vi "顺序结构.vi"() -> ()   [LabVIEW 2017]
panel:
  out "布尔":bool
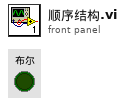
[diagram p1: front panel]
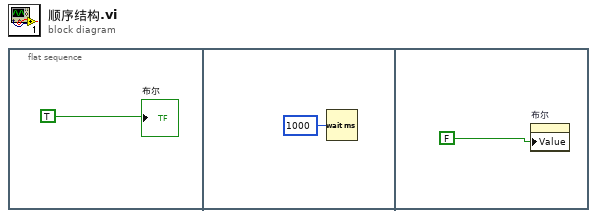
[diagram p0: block diagram]
diagram:
  n1 = flat-sequence {
    frame #0 {
      "布尔" <- TRUE
    }
    frame #1 {
      n2 = Wait (ms)(milliseconds to wait=u32 1000 ("等待时间（毫秒）")) -> ()  [unwired: 1 out]
    }
    frame #2 {
      n3 = property on="布尔" class="Bool (严格)"("Value"=FALSE) -> ()  [unwired: 2 in, 2 out]
    }
  }
